vi "GeoData.vi"() -> ()   [LabVIEW 2017] (continued)
NJ\tBurlington County\tH1\n8022\t34005\tColumbus\tNJ\tBurlington County\tH1\n8060\t34005\tMount holly\tNJ\tBurlington County\tH1\n8640\t34005\tJoint base mdl\tNJ\tBurlington County\tH1\n8073\t34005\tRancocas\tNJ\tBurlington County\tH1\n8224\t34005\tNew gretna\tNJ\tBurlington County\tH1\n8043\t34005\tVoorhees\tNJ\tBurlington County\tH1\n8065\t34005\tPalmyra\tNJ\tBurlington County\tH1\n8052\t34005\tMaple shade\tNJ\tBurlington County\tH1\n8515\t34005\tChesterfield\tNJ\tBurlington County\tH1\n8046\t34005\tWillingboro\tNJ\tBurlington County\tH1\n8077\t34005\tRiverton\tNJ\tBurlington County\tH1\n8091\t34005\tWest berlin\tNJ\tBurlington County\tH1\n8641\t34005\tJoint base mdl\tNJ\tBurlington County\tH1\n8041\t34005\tJobstown\tNJ\tBurlington County\tH1\n8064\t34005\tNew lisbon\tNJ\tBurlington County\tH1\n8015\t34005\tBrowns mills\tNJ\tBurlington County\tH1\n8057\t34005\tMoorestown\tNJ\tBurlington County\tH1\n8087\t34005\tTuckerton\tNJ\tBurlington County\tH1\n8110\t34005\tPennsauken\tNJ\tBurlington County\tH1\n8215\t34005\tEgg harbor city\tNJ\tBurlington County\tH1\n8518\t34005\tFlorence\tNJ\tBurlington County\tH1\n8042\t34005\tJuliustown\tNJ\tBurlington County\tH1\n8053\t34005\tMarlton\tNJ\tBurlington County\tH1\n8054\t34005\tMount laurel\tNJ\tBurlington County\tH1\n8075\t34005\tRiverside\tNJ\tBurlington County\tH1\n8562\t34005\tWrightstown\tNJ\tBurlington County\tH1\n8620\t34005\tTrenton\tNJ\tBurlington County\tH1\n8011\t34005\tBirmingham\tNJ\tBurlington County\tH1\n8004\t34005\tAtco\tNJ\tBurlington County\tH1\n8010\t34005\tBeverly\tNJ\tBurlington County\tH1\n8048\t34005\tLumberton\tNJ\tBurlington County\tH1\n8088\t34005\tVincentown\tNJ\tBurlington County\tH1\n8068\t34005\tPemberton\tNJ\tBurlington County\tH1\n8016\t34005\tBurlington\tNJ\tBurlington County\tH1\n8055\t34005\tMedford\tNJ\tBurlington County\tH1\n8511\t34005\tCookstown\tNJ\tBurlington County\tH1\n8554\t34005\tRoebling\tNJ\tBurlington County\tH1\n8012\t34007\tBlackwood\tNJ\tCamden County\tH1\n8109\t34007\tMerchantville\tNJ\tCamden County\tH1\n8108\t34007\tCollingswood\tNJ\tCamden County\tH1\n8029\t34007\tGlendora\tNJ\tCamden County\tH1\n8002\t34007\tCherry hill\tNJ\tCamden County\tH1\n8037\t34007\tHammonton\tNJ\tCamden County\tH1\n8033\t34007\tHaddonfield\tNJ\tCamden County\tH1\n8049\t34007\tMagnolia\tNJ\tCamden County\tH1\n8081\t34007\tSicklerville\tNJ\tCamden County\tH1\n8035\t34007\tHaddon heights\tNJ\tCamden County\tH1\n8009\t34007\tBerlin\tNJ\tCamden County\tH1\n8043\t34007\tVoorhees\tNJ\tCamden County\tH1\n8065\t34007\tPalmyra\tNJ\tCamden County\tH1\n8052\t34007\tMaple shade\tNJ\tCamden County\tH1\n8080\t34007\tSewell\tNJ\tCamden County\tH1\n8084\t34007\tStratford\tNJ\tCamden County\tH1\n8106\t34007\tAudubon\tNJ\tCamden County\tH1\n8105\t34007\tCamden\tNJ\tCamden County\tH1\n8101\t34007\tCamden\tNJ\tCamden County\tH1\n8003\t34007\tCherry hill\tNJ\tCamden County\tH1\n8021\t34007\tClementon\tNJ\tCamden County\tH1\n8030\t34007\tGloucester city\tNJ\tCamden County\tH1\n8083\t34007\tSomerdale\tNJ\tCamden County\tH1\n8103\t34007\tCamden\tNJ\tCamden County\tH1\n8091\t34007\tWest berlin\tNJ\tCamden County\tH1\n8102\t34007\tCamden\tNJ\tCamden County\tH1\n8045\t34007\tLawnside\tNJ\tCamden County\tH1\n8110\t34007\tPennsauken\tNJ\tCamden County\tH1\n8099\t34007\tBellmawr\tNJ\tCamden County\tH1\n8095\t34007\tWinslow\tNJ\tCamden County\tH1\n8018\t34007\tCedar brook\tNJ\tCamden County\tH1\n8007\t34007\tBarrington\tNJ\tCamden County\tH1\n8026\t34007\tGibbsboro\tNJ\tCamden County\tH1\n8078\t34007\tRunnemede\tNJ\tCamden County\tH1\n8004\t34007\tAtco\tNJ\tCamden County\tH1\n8034\t34007\tCherry hill\tNJ\tCamden County\tH1\n8107\t34007\tOaklyn\tNJ\tCamden County\tH1\n8059\t34007\tMount ephraim\tNJ\tCamden County\tH1\n8104\t34007\tCamden\tNJ\tCamden County\tH1\n8089\t34007\tWaterford works\tNJ\tCamden County\tH1\n8031\t34007\tBellmawr\tNJ\tCamden County\tH1\n8223\t34009\tMarmora\tNJ\tCape May County\tH1\n8212\t34009\tCape may point\tNJ\tCape May County\tH1\n8248\t34009\tStrathmere\tNJ\tCape May County\tH1\n8260\t34009\tWildwood\tNJ\tCape May County\tH1\n8270\t34009\tWoodbine\tNJ\tCape May County\tH1\n8245\t34009\tSouth dennis\tNJ\tCape May County\tH1\n8204\t34009\tCape may\tNJ\tCape May County\tH1\n8202\t34009\tAvalon\tNJ\tCape May County\tH1\n8230\t34009\tOcean view\tNJ\tCape May County\tH1\n8214\t34009\tDennisville\tNJ\tCape May County\tH1\n8218\t34009\tGoshen\tNJ\tCape May County\tH1\n8210\t34009\tCape may court house\tNJ\tCape May County\tH1\n8246\t34009\tSouth seaville\tNJ\tCape May County\tH1\n8247\t34009\tStone harbor\tNJ\tCape May County\tH1\n8314\t34009\tDelmont\tNJ\tCape May County\tH1\n8226\t34009\tOcean city\tNJ\tCape May County\tH1\n8252\t34009\tWhitesboro\tNJ\tCape May County\tH1\n8251\t34009\tVillas\tNJ\tCape May County\tH1\n8242\t34009\tRio grande\tNJ\tCape May County\tH1\n8250\t34009\tTuckahoe\tNJ\tCape May County\tH1\n8243\t34009\tSea isle city\tNJ\tCape May County\tH1\n8219\t34009\tGreen creek\tNJ\tCape May County\tH1\n8353\t34011\tShiloh\tNJ\tCumberland County\tH1\n8340\t34011\tMilmay\tNJ\tCumberland County\tH1\n8324\t34011\tHeislerville\tNJ\tCumberland County\tH1\n8313\t34011\tDeerfield street\tNJ\tCumberland County\tH1\n8332\t34011\tMillville\tNJ\tCumberland County\tH1\n8302\t34011\tBridgeton\tNJ\tCumberland County\tH1\n8270\t34011\tWoodbine\tNJ\tCumberland County\tH1\n8361\t34011\tVineland\tNJ\tCumberland County\tH1\n8321\t34011\tFortescue\tNJ\tCumberland County\tH1\n8320\t34011\tFairton\tNJ\tCumberland County\tH1\n8345\t34011\tNewport\tNJ\tCumberland County\tH1\n8329\t34011\tMauricetown\tNJ\tCumberland County\tH1\n8311\t34011\tCedarville\tNJ\tCumberland County\tH1\n8349\t34011\tPort norris\tNJ\tCumberland County\tH1\n8348\t34011\tPort elizabeth\tNJ\tCumberland County\tH1\n8316\t34011\tDorchester\tNJ\tCumberland County\tH1\n8360\t34011\tVineland\tNJ\tCumberland County\tH1\n8314\t34011\tDelmont\tNJ\tCumberland County\tH1\n8327\t34011\tLeesburg\tNJ\tCumberland County\tH1\n8352\t34011\tRosenhayn\tNJ\tCumberland County\tH1\n8318\t34011\tElmer\tNJ\tCumberland County\tH1\n8310\t34011\tBuena\tNJ\tCumberland County\tH1\n8315\t34011\tDividing creek\tNJ\tCumberland County\tH1\n8323\t34011\tGreenwich\tNJ\tCumberland County\tH1\n8344\t34011\tNewfield\tNJ\tCumberland County\tH1\n8362\t34011\tVineland\tNJ\tCumberland County\tH1\n7040\t34013\tMaplewood\tNJ\tEssex County\tH1\n7052\t34013\tWest orange\tNJ\tEssex County\tH1\n7068\t34013\tRoseland\tNJ\tEssex County\tH1\n7102\t34013\tNewark\tNJ\tEssex County\tH1\n7114\t34013\tNewark\tNJ\tEssex County\tH1\n7108\t34013\tNewark\tNJ\tEssex County\tH1\n7109\t34013\tBelleville\tNJ\tEssex County\tH1\n7107\t34013\tNewark\tNJ\tEssex County\tH1\n7003\t34013\tBloomfield\tNJ\tEssex County\tH1\n7021\t34013\tEssex fells\tNJ\tEssex County\tH1\n7042\t34013\tMontclair\tNJ\tEssex County\tH1\n7106\t34013\tNewark\tNJ\tEssex County\tH1\n7044\t34013\tVerona\tNJ\tEssex County\tH1\n7050\t34013\tOrange\tNJ\tEssex County\tH1\n7104\t34013\tNewark\tNJ\tEssex County\tH1\n7101\t34013\tNewark\tNJ\tEssex County\tH1\n7088\t34013\tVauxhall\tNJ\tEssex County\tH1\n7009\t34013\tCedar grove\tNJ\tEssex County\tH1\n7039\t34013\tLivingston\tNJ\tEssex County\tH1\n7111\t34013\tIrvington\tNJ\tEssex County\tH1\n7201\t34013\tElizabeth\tNJ\tEssex County\tH1\n7017\t34013\tEast orange\tNJ\tEssex County\tH1\n7004\t34013\tFairfield\tNJ\tEssex County\tH1\n7041\t34013\tMillburn\tNJ\tEssex County\tH1\n7175\t34013\tNewark\tNJ\tEssex County\tH1\n7083\t34013\tUnion\tNJ\tEssex County\tH1\n7007\t34013\tCaldwell\tNJ\tEssex County\tH1\n7051\t34013\tOrange\tNJ\tEssex County\tH1\n7018\t34013\tEast orange\tNJ\tEssex County\tH1\n7043\t34013\tMontclair\tNJ\tEssex County\tH1\n7079\t34013\tSouth orange\tNJ\tEssex County\tH1\n7103\t34013\tNewark\tNJ\tEssex County\tH1\n7112\t34013\tNewark\tNJ\tEssex County\tH1\n7205\t34013\tHillside\tNJ\tEssex County\tH1\n7028\t34013\tGlen ridge\tNJ\tEssex County\tH1\n7006\t34013\tCaldwell\tNJ\tEssex County\tH1\n7019\t34013\tEast orange\tNJ\tEssex County\tH1\n7078\t34013\tShort hills\tNJ\tEssex County\tH1\n7110\t34013\tNutley\tNJ\tEssex County\tH1\n7105\t34013\tNewark\tNJ\tEssex County\tH1\n8012\t34015\tBlackwood\tNJ\tGloucester County\tH1\n8051\t34015\tMantua\tNJ\tGloucester County\tH1\n8098\t34015\tWoodstown\tNJ\tGloucester County\tH1\n8328\t34015\tMalaga\tNJ\tGloucester County\tH1\n8061\t34015\tMount royal\tNJ\tGloucester County\tH1\n8081\t34015\tSicklerville\tNJ\tGloucester County\tH1\n8085\t34015\tSwedesboro\tNJ\tGloucester County\tH1\n8096\t34015\tWoodbury\tNJ\tGloucester County\tH1\n8322\t34015\tFranklinville\tNJ\tGloucester County\tH1\n8312\t34015\tClayton\tNJ\tGloucester County\tH1\n8074\t34015\tRichwood\tNJ\tGloucester County\tH1\n8080\t34015\tSewell\tNJ\tGloucester County\tH1\n8071\t34015\tPitman\tNJ\tGloucester County\tH1\n8028\t34015\tGlassboro\tNJ\tGloucester County\tH1\n8063\t34015\tNational park\tNJ\tGloucester County\tH1\n8086\t34015\tThorofare\tNJ\tGloucester County\tH1\n8093\t34015\tWestville\tNJ\tGloucester County\tH1\n8097\t34015\tWoodbury heights\tNJ\tGloucester County\tH1\n8056\t34015\tMickleton\tNJ\tGloucester County\tH1\n8014\t34015\tBridgeport\tNJ\tGloucester County\tH1\n8094\t34015\tWilliamstown\tNJ\tGloucester County\tH1\n8360\t34015\tVineland\tNJ\tGloucester County\tH1\n8062\t34015\tMullica hill\tNJ\tGloucester County\tH1\n8343\t34015\tMonroeville\tNJ\tGloucester County\tH1\n8025\t34015\tEwan\tNJ\tGloucester County\tH1\n8020\t34015\tClarksboro\tNJ\tGloucester County\tH1\n8066\t34015\tPaulsboro\tNJ\tGloucester County\tH1\n8090\t34015\tWenonah\tNJ\tGloucester County\tH1\n8032\t34015\tGrenloch\tNJ\tGloucester County\tH1\n8027\t34015\tGibbstown\tNJ\tGloucester County\tH1\n8344\t34015\tNewfield\tNJ\tGloucester County\tH1\n8039\t34015\tHarrisonville\tNJ\tGloucester County\tH1\n7303\t34017\tJersey city\tNJ\tHudson County\tH1\n7087\t34017\tUnion city\tNJ\tHudson County\tH1\n7310\t34017\tJersey city\tNJ\tHudson County\tH1\n7002\t34017\tBayonne\tNJ\tHudson County\tH1\n7031\t34017\tNorth arlington\tNJ\tHudson County\tH1\n7047\t34017\tNorth bergen\tNJ\tHudson County\tH1\n7302\t34017\tJersey city\tNJ\tHudson County\tH1\n7311\t34017\tJersey city\tNJ\tHudson County\tH1\n7097\t34017\tJersey city\tNJ\tHudson County\tH1\n7093\t34017\tWest new york\tNJ\tHudson County\tH1\n7304\t34017\tJersey city\tNJ\tHudson County\tH1\n7030\t34017\tHoboken\tNJ\tHudson County\tH1\n7094\t34017\tSecaucus\tNJ\tHudson County\tH1\n7307\t34017\tJersey city\tNJ\tHudson County\tH1\n7096\t34017\tSecaucus\tNJ\tHudson County\tH1\n7099\t34017\tKearny\tNJ\tHudson County\tH1\n7032\t34017\tKearny\tNJ\tHudson County\tH1\n7029\t34017\tHarrison\tNJ\tHudson County\tH1\n7086\t34017\tWeehawken\tNJ\tHudson County\tH1\n7305\t34017\tJersey city\tNJ\tHudson County\tH1\n7306\t34017\tJersey city\tNJ\tHudson County\tH1\n7399\t34017\tJersey city\tNJ\tHudson County\tH1\n8833\t34019\tLebanon\tNJ\tHunterdon County\tH1\n7865\t34019\tPort murray\tNJ\tHunterdon County\tH1\n8801\t34019\tAnnandale\tNJ\tHunterdon County\tH1\n8559\t34019\tStockton\tNJ\tHunterdon County\tH1\n8551\t34019\tRingoes\tNJ\tHunterdon County\tH1\n7831\t34019\tChangewater\tNJ\tHunterdon County\tH1\n8803\t34019\tBaptistown\tNJ\tHunterdon County\tH1\n7830\t34019\tCalifon\tNJ\tHunterdon County\tH1\n8802\t34019\tAsbury\tNJ\tHunterdon County\tH1\n8558\t34019\tSkillman\tNJ\tHunterdon County\tH1\n8825\t34019\tFrenchtown\tNJ\tHunterdon County\tH1\n8848\t34019\tMilford\tNJ\tHunterdon County\tH1\n8804\t34019\tBloomsbury\tNJ\tHunterdon County\tH1\n8887\t34019\tThree bridges\tNJ\tHunterdon County\tH1\n8885\t34019\tStanton\tNJ\tHunterdon County\tH1\n8876\t34019\tSomerville\tNJ\tHunterdon County\tH1\n8530\t34019\tLambertville\tNJ\tHunterdon County\tH1\n8809\t34019\tClinton\tNJ\tHunterdon County\tH1\n8525\t34019\tHopewell\tNJ\tHunterdon County\tH1\n8867\t34019\tPittstown\tNJ\tHunterdon County\tH1\n8560\t34019\tTitusville\tNJ\tHunterdon County\tH1\n8868\t34019\tQuakertown\tNJ\tHunterdon County\tH1\n8888\t34019\tWhitehouse\tNJ\tHunterdon County\tH1\n7882\t34019\tWashington\tNJ\tHunterdon County\tH1\n8822\t34019\tFlemington\tNJ\tHunterdon County\tH1\n8889\t34019\tWhitehouse station\tNJ\tHunterdon County\tH1\n8827\t34019\tHampton\tNJ\tHunterdon County\tH1\n8556\t34019\tRosemont\tNJ\tHunterdon County\tH1\n8870\t34019\tReadington\tNJ\tHunterdon County\tH1\n8557\t34019\tSergeantsville\tNJ\tHunterdon County\tH1\n8829\t34019\tHigh bridge\tNJ\tHunterdon County\tH1\n8826\t34019\tGlen gardner\tNJ\tHunterdon County\tH1\n8858\t34019\tOldwick\tNJ\tHunterdon County\tH1\n8853\t34019\tNeshanic station\tNJ\tHunterdon County\tH1\n7979\t34019\tPottersville\tNJ\tHunterdon County\tH1\n8512\t34021\tCranbury\tNJ\tMercer County\tH1\n8501\t34021\tAllentown\tNJ\tMercer County\tH1\n8610\t34021\tTrenton\tNJ\tMercer County\tH1\n8542\t34021\tPrinceton\tNJ\tMercer County\tH1\n8628\t34021\tTrenton\tNJ\tMercer County\tH1\n8604\t34021\tTrenton\tNJ\tMercer County\tH1\n8601\t34021\tTrenton\tNJ\tMercer County\tH1\n8534\t34021\tPennington\tNJ\tMercer County\tH1\n8607\t34021\tTrenton\tNJ\tMercer County\tH1\n8540\t34021\tPrinceton\tNJ\tMercer County\tH1\n8558\t34021\tSkillman\tNJ\tMercer County\tH1\n8638\t34021\tTrenton\tNJ\tMercer County\tH1\n8648\t34021\tLawrence township\tNJ\tMercer County\tH1\n8515\t34021\tChesterfield\tNJ\tMercer County\tH1\n8543\t34021\tPrinceton\tNJ\tMercer County\tH1\n8602\t34021\tTrenton\tNJ\tMercer County\tH1\n8550\t34021\tPrinceton junction\tNJ\tMercer County\tH1\n8629\t34021\tTrenton\tNJ\tMercer County\tH1\n8544\t34021\tPrinceton\tNJ\tMercer County\tH1\n8530\t34021\tLambertville\tNJ\tMercer County\tH1\n8561\t34021\tWindsor\tNJ\tMercer County\tH1\n8520\t34021\tHightstown\tNJ\tMercer County\tH1\n8691\t34021\tTrenton\tNJ\tMercer County\tH1\n8618\t34021\tTrenton\tNJ\tMercer County\tH1\n8650\t34021\tTrenton\tNJ\tMercer County\tH1\n8606\t34021\tTrenton\tNJ\tMercer County\tH1\n8603\t34021\tTrenton\tNJ\tMercer County\tH1\n8608\t34021\tTrenton\tNJ\tMercer County\tH1\n8525\t34021\tHopewell\tNJ\tMercer County\tH1\n8619\t34021\tTrenton\tNJ\tMercer County\tH1\n8690\t34021\tTrenton\tNJ\tMercer County\tH1\n8620\t34021\tTrenton\tNJ\tMercer County\tH1\n8560\t34021\tTitusville\tNJ\tMercer County\tH1\n8605\t34021\tTrenton\tNJ\tMercer County\tH1\n8609\t34021\tTrenton\tNJ\tMercer County\tH1\n8611\t34021\tTrenton\tNJ\tMercer County\tH1\n8902\t34023\tNorth brunswick\tNJ\tMiddlesex County\tH1\n8882\t34023\tSouth river\tNJ\tMiddlesex County\tH1\n8512\t34023\tCranbury\tNJ\tMiddlesex County\tH1\n7067\t34023\tColonia\tNJ\tMiddlesex County\tH1\n7064\t34023\tPort reading\tNJ\tMiddlesex County\tH1\n8812\t34023\tDunellen\tNJ\tMiddlesex County\tH1\n7735\t34023\tKeyport\tNJ\tMiddlesex County\tH1\n8536\t34023\tPlainsboro\tNJ\tMiddlesex County\tH1\n8828\t34023\tHelmetta\tNJ\tMiddlesex County\tH1\n8903\t34023\tNew brunswick\tNJ\tMiddlesex County\tH1\n7008\t34023\tCarteret\tNJ\tMiddlesex County\tH1\n8816\t34023\tEast brunswick\tNJ\tMiddlesex County\tH1\n8830\t34023\tIselin\tNJ\tMiddlesex County\tH1\n8832\t34023\tKeasbey\tNJ\tMiddlesex County\tH1\n8857\t34023\tOld bridge\tNJ\tMiddlesex County\tH1\n7747\t34023\tMatawan\tNJ\tMiddlesex County\tH1\n8540\t34023\tPrinceton\tNJ\tMiddlesex County\tH1\n8863\t34023\tFords\tNJ\tMiddlesex County\tH1\n8855\t34023\tPiscataway\tNJ\tMiddlesex County\tH1\n8933\t34023\tNew brunswick\tNJ\tMiddlesex County\tH1\n7001\t34023\tAvenel\tNJ\tMiddlesex County\tH1\n8817\t34023\tEdison\tNJ\tMiddlesex County\tH1\n8820\t34023\tEdison\tNJ\tMiddlesex County\tH1\n8862\t34023\tPerth amboy\tNJ\tMiddlesex County\tH1\n8884\t34023\tSpotswood\tNJ\tMiddlesex County\tH1\n7095\t34023\tWoodbridge\tNJ\tMiddlesex County\tH1\n8810\t34023\tDayton\tNJ\tMiddlesex County\tH1\n8818\t34023\tEdison\tNJ\tMiddlesex County\tH1\n8852\t34023\tMonmouth junction\tNJ\tMiddlesex County\tH1\n8859\t34023\tParlin\tNJ\tMiddlesex County\tH1\n8904\t34023\tHighland park\tNJ\tMiddlesex County\tH1\n8520\t34023\tHightstown\tNJ\tMiddlesex County\tH1\n8805\t34023\tBound brook\tNJ\tMiddlesex County\tH1\n8854\t34023\tPiscataway\tNJ\tMiddlesex County\tH1\n8879\t34023\tSouth amboy\tNJ\tMiddlesex County\tH1\n7065\t34023\tRahway\tNJ\tMiddlesex County\tH1\n7080\t34023\tSouth plainfield\tNJ\tMiddlesex County\tH1\n8823\t34023\tFranklin park\tNJ\tMiddlesex County\tH1\n8824\t34023\tKendall park\tNJ\tMiddlesex County\tH1\n8850\t34023\tMilltown\tNJ\tMiddlesex County\tH1\n8861\t34023\tPerth amboy\tNJ\tMiddlesex County\tH1\n8872\t34023\tSayreville\tNJ\tMiddlesex County\tH1\n8901\t34023\tNew brunswick\tNJ\tMiddlesex County\tH1\n7721\t34023\tCliffwood\tNJ\tMiddlesex County\tH1\n7751\t34023\tMorganville\tNJ\tMiddlesex County\tH1\n7077\t34023\tSewaren\tNJ\tMiddlesex County\tH1\n8831\t34023\tMonroe township\tNJ\tMiddlesex County\tH1\n8840\t34023\tMetuchen\tNJ\tMiddlesex County\tH1\n8846\t34023\tMiddlesex\tNJ\tMiddlesex County\tH1\n8837\t34023\tEdison\tNJ\tMiddlesex County\tH1\n7726\t34023\tEnglishtown\tNJ\tMiddlesex County\tH1\n8528\t34023\tKingston\tNJ\tMiddlesex County\tH1\n8906\t34023\tNew brunswick\tNJ\tMiddlesex County\tH1\n8899\t34023\tEdison\tNJ\tMiddlesex County\tH1\n7727\t34025\tFarmingdale\tNJ\tMonmouth County\tH1\n7723\t34025\tDeal\tNJ\tMonmouth County\tH1\n7738\t34025\tLincroft\tNJ\tMonmouth County\tH1\n7754\t34025\tNeptune\tNJ\tMonmouth County\tH1\n7739\t34025\tLittle silver\tNJ\tMonmouth County\tH1\n8501\t34025\tAllentown\tNJ\tMonmouth County\tH1\n8736\t34025\tManasquan\tNJ\tMonmouth County\tH1\n7718\t34025\tBelford\tNJ\tMonmouth County\tH1\n7701\t34025\tRed bank\tNJ\tMonmouth County\tH1\n7712\t34025\tAsbury park\tNJ\tMonmouth County\tH1\n7732\t34025\tHighlands\tNJ\tMonmouth County\tH1\n7760\t34025\tRumson\tNJ\tMonmouth County\tH1\n7735\t34025\tKeyport\tNJ\tMonmouth County\tH1\n7764\t34025\tWest long branch\tNJ\tMonmouth County\tH1\n8514\t34025\tCream ridge\tNJ\tMonmouth County\tH1\n8527\t34025\tJackson\tNJ\tMonmouth County\tH1\n8750\t34025\tSea girt\tNJ\tMonmouth County\tH1\n7752\t34025\tNavesink\tNJ\tMonmouth County\tH1\n8555\t34025\tRoosevelt\tNJ\tMonmouth County\tH1\n7704\t34025\tFair haven\tNJ\tMonmouth County\tH1\n7728\t34025\tFreehold\tNJ\tMonmouth County\tH1\n7747\t34025\tMatawan\tNJ\tMonmouth County\tH1\n7746\t34025\tMarlboro\tNJ\tMonmouth County\tH1\n7762\t34025\tSpring lake\tNJ\tMonmouth County\tH1\n8730\t34025\tBrielle\tNJ\tMonmouth County\tH1\n7711\t34025\tAllenhurst\tNJ\tMonmouth County\tH1\n7710\t34025\tAdelphia\tNJ\tMonmouth County\tH1\n7731\t34025\tHowell\tNJ\tMonmouth County\tH1\n7740\t34025\tLong branch\tNJ\tMonmouth County\tH1\n7748\t34025\tMiddletown\tNJ\tMonmouth County\tH1\n8720\t34025\tAllenwood\tNJ\tMonmouth County\tH1\n7703\t34025\tFort monmouth\tNJ\tMonmouth County\tH1\n7733\t34025\tHolmdel\tNJ\tMonmouth County\tH1\n7719\t34025\tBelmar\tNJ\tMonmouth County\tH1\n7750\t34025\tMonmouth beach\tNJ\tMonmouth County\tH1\n8520\t34025\tHightstown\tNJ\tMonmouth County\tH1\n8535\t34025\tMillstone township\tNJ\tMonmouth County\tH1\n8691\t34025\tTrenton\tNJ\tMonmouth County\tH1\n7763\t34025\tTennent\tNJ\tMonmouth County\tH1\n7799\t34025\tEatontown\tNJ\tMonmouth County\tH1\n7724\t34025\tEatontown\tNJ\tMonmouth County\tH1\n7730\t34025\tHazlet\tNJ\tMonmouth County\tH1\n7737\t34025\tLeonardo\tNJ\tMonmouth County\tH1\n7757\t34025\tOceanport\tNJ\tMonmouth County\tH1\n7758\t34025\tPort monmouth\tNJ\tMonmouth County\tH1\n8562\t34025\tWrightstown\tNJ\tMonmouth County\tH1\n8620\t34025\tTrenton\tNJ\tMonmouth County\tH1\n7720\t34025\tBradley beach\tNJ\tMonmouth County\tH1\n7765\t34025\tWickatunk\tNJ\tMonmouth County\tH1\n7716\t34025\tAtlantic highlands\tNJ\tMonmouth County\tH1\n7721\t34025\tCliffwood\tNJ\tMonmouth County\tH1\n7751\t34025\tMorganville\tNJ\tMonmouth County\tH1\n7753\t34025\tNeptune\tNJ\tMonmouth County\tH1\n8510\t34025\tMillstone township\tNJ\tMonmouth County\tH1\n7755\t34025\tOakhurst\tNJ\tMonmouth County\tH1\n7702\t34025\tShrewsbury\tNJ\tMonmouth County\tH1\n7717\t34025\tAvon by the sea\tNJ\tMonmouth County\tH1\n7726\t34025\tEnglishtown\tNJ\tMonmouth County\tH1\n7734\t34025\tKeansburg\tNJ\tMonmouth County\tH1\n7722\t34025\tColts neck\tNJ\tMonmouth County\tH1\n7756\t34025\tOcean grove\tNJ\tMonmouth County\tH1\n8724\t34025\tBrick\tNJ\tMonmouth County\tH1\n7927\t34027\tCedar knolls\tNJ\tMorris County\tH1\n7457\t34027\tRiverdale\tNJ\tMorris County\tH1\n7935\t34027\tGreen village\tNJ\tMorris County\tH1\n7082\t34027\tTowaco\tNJ\tMorris County\tH1\n7405\t34027\tButler\tNJ\tMorris County\tH1\n7852\t34027\tLedgewood\tNJ\tMorris County\tH1\n7849\t34027\tLake hopatcong\tNJ\tMorris County\tH1\n7865\t34027\tPort murray\tNJ\tMorris County\tH1\n7936\t34027\tEast hanover\tNJ\tMorris County\tH1\n7933\t34027\tGillette\tNJ\tMorris County\tH1\n7932\t34027\tFlorham park\tNJ\tMorris County\tH1\n7930\t34027\tChester\tNJ\tMorris County\tH1\n7970\t34027\tMount freedom\tNJ\tMorris County\tH1\n7054\t34027\tParsippany\tNJ\tMorris County\tH1\n7403\t34027\tBloomingdale\tNJ\tMorris County\tH1\n7828\t34027\tBudd lake\tNJ\tMorris County\tH1\n7836\t34027\tFlanders\tNJ\tMorris County\tH1\n7830\t34027\tCalifon\tNJ\tMorris County\tH1\n7976\t34027\tNew vernon\tNJ\tMorris County\tH1\n7962\t34027\tMorristown\tNJ\tMorris County\tH1\n7058\t34027\tPine brook\tNJ\tMorris County\tH1\n7801\t34027\tDover\tNJ\tMorris County\tH1\n7850\t34027\tLanding\tNJ\tMorris County\tH1\n7866\t34027\tRockaway\tNJ\tMorris County\tH1\n7945\t34027\tMendham\tNJ\tMorris County\tH1\n7878\t34027\tMount tabor\tNJ\tMorris County\tH1\n7870\t34027\tSchooleys mountain\tNJ\tMorris County\tH1\n7034\t34027\tLake hiawatha\tNJ\tMorris County\tH1\n7940\t34027\tMadison\tNJ\tMorris County\tH1\n7926\t34027\tBrookside\tNJ\tMorris County\tH1\n7961\t34027\tConvent station\tNJ\tMorris County\tH1\n7845\t34027\tIronia\tNJ\tMorris County\tH1\n7005\t34027\tBoonton\tNJ\tMorris County\tH1\n7460\t34027\tStockholm\tNJ\tMorris County\tH1\n7834\t34027\tDenville\tNJ\tMorris County\tH1\n7856\t34027\tMount arlington\tNJ\tMorris County\tH1\n7847\t34027\tKenvil\tNJ\tMorris County\tH1\n7928\t34027\tChatham\tNJ\tMorris County\tH1\n7885\t34027\tWharton\tNJ\tMorris County\tH1\n7980\t34027\tStirling\tNJ\tMorris County\tH1\n7802\t34027\tDover\tNJ\tMorris County\tH1\n7857\t34027\tNetcong\tNJ\tMorris County\tH1\n7035\t34027\tLincoln park\tNJ\tMorris County\tH1\n7045\t34027\tMontville\tNJ\tMorris County\tH1\n7444\t34027\tPompton plains\tNJ\tMorris County\tH1\n7438\t34027\tOak ridge\tNJ\tMorris County\tH1\n7803\t34027\tMine hill\tNJ\tMorris County\tH1\n7869\t34027\tRandolph\tNJ\tMorris County\tH1\n7920\t34027\tBasking ridge\tNJ\tMorris County\tH1\n7960\t34027\tMorristown\tNJ\tMorris County\tH1\n7950\t34027\tMorris plains\tNJ\tMorris County\tH1\n7931\t34027\tFar hills\tNJ\tMorris County\tH1\n7924\t34027\tBernardsville\tNJ\tMorris County\tH1\n7981\t34027\tWhippany\tNJ\tMorris County\tH1\n7046\t34027\tMountain lakes\tNJ\tMorris County\tH1\n7963\t34027\tMorristown\tNJ\tMorris County\tH1\n7435\t34027\tNewfoundland\tNJ\tMorris County\tH1\n7853\t34027\tLong valley\tNJ\tMorris County\tH1\n7840\t34027\tHackettstown\tNJ\tMorris County\tH1\n7876\t34027\tSuccasunna\tNJ\tMorris County\tH1\n7946\t34027\tMillington\tNJ\tMorris County\tH1\n7934\t34027\tGladstone\tNJ\tMorris County\tH1\n7440\t34027\tPequannock\tNJ\tMorris County\tH1\n7806\t34027\tPicatinny arsenal\tNJ\tMorris County\tH1\n7842\t34027\tHibernia\tNJ\tMorris County\tH1\n8734\t34029\tLanoka harbor\tNJ\tOcean County\tH1\n8757\t34029\tToms river\tNJ\tOcean County\tH1\n8759\t34029\tManchester township\tNJ\tOcean County\tH1\n8758\t34029\tWaretown\tNJ\tOcean County\tH1\n8754\t34029\tToms river\tNJ\tOcean County\tH1\n8514\t34029\tCream ridge\tNJ\tOcean County\tH1\n8527\t34029\tJackson\tNJ\tOcean County\tH1\n8753\t34029\tToms river\tNJ\tOcean County\tH1\n8741\t34029\tPine beach\tNJ\tOcean County\tH1\n8739\t34029\tNormandy beach\tNJ\tOcean County\tH1\n7728\t34029\tFreehold\tNJ\tOcean County\tH1\n8006\t34029\tBarnegat light\tNJ\tOcean County\tH1\n7731\t34029\tHowell\tNJ\tOcean County\tH1\n8721\t34029\tBayville\tNJ\tOcean County\tH1\n8723\t34029\tBrick\tNJ\tOcean County\tH1\n8733\t34029\tLakehurst\tNJ\tOcean County\tH1\n8087\t34029\tTuckerton\tNJ\tOcean County\tH1\n8722\t34029\tBeachwood\tNJ\tOcean County\tH1\n8742\t34029\tPoint pleasant beach\tNJ\tOcean County\tH1\n8751\t34029\tSeaside heights\tNJ\tOcean County\tH1\n8731\t34029\tForked river\tNJ\tOcean County\tH1\n8752\t34029\tSeaside park\tNJ\tOcean County\tH1\n8732\t34029\tIsland heights\tNJ\tOcean County\tH1\n8701\t34029\tLakewood\tNJ\tOcean County\tH1\n8533\t34029\tNew egypt\tNJ\tOcean County\tH1\n8008\t34029\tBeach haven\tNJ\tOcean County\tH1\n8050\t34029\tManahawkin\tNJ\tOcean County\tH1\n8735\t34029\tLavallette\tNJ\tOcean County\tH1\n8740\t34029\tOcean gate\tNJ\tOcean County\tH1\n8755\t34029\tToms river\tNJ\tOcean County\tH1\n8005\t34029\tBarnegat\tNJ\tOcean County\tH1\n8092\t34029\tWest creek\tNJ\tOcean County\tH1\n8724\t34029\tBrick\tNJ\tOcean County\tH1\n8738\t34029\tMantoloking\tNJ\tOcean County\tH1\n7013\t34031\tClifton\tNJ\tPassaic County\tH1\n7012\t34031\tClifton\tNJ\tPassaic County\tH1\n7424\t34031\tLittle falls\tNJ\tPassaic County\tH1\n7508\t34031\tHaledon\tNJ\tPassaic County\tH1\n7522\t34031\tPaterson\tNJ\tPassaic County\tH1\n7474\t34031\tWayne\tNJ\tPassaic County\tH1\n7503\t34031\tPaterson\tNJ\tPassaic County\tH1\n7015\t34031\tClifton\tNJ\tPassaic County\tH1\n7421\t34031\tHewitt\tNJ\tPassaic County\tH1\n7403\t34031\tBloomingdale\tNJ\tPassaic County\tH1\n7506\t34031\tHawthorne\tNJ\tPassaic County\tH1\n7481\t34031\tWyckoff\tNJ\tPassaic County\tH1\n7507\t34031\tHawthorne\tNJ\tPassaic County\tH1\n7055\t34031\tPassaic\tNJ\tPassaic County\tH1\n7501\t34031\tPaterson\tNJ\tPassaic County\tH1\n7512\t34031\tTotowa\tNJ\tPassaic County\tH1\n7480\t34031\tWest milford\tNJ\tPassaic County\tH1\n7505\t34031\tPaterson\tNJ\tPassaic County\tH1\n7511\t34031\tTotowa\tNJ\tPassaic County\tH1\n7538\t34031\tHaledon\tNJ\tPassaic County\tH1\n7543\t34031\tPaterson\tNJ\tPassaic County\tH1\n7504\t34031\tPaterson\tNJ\tPassaic County\tH1\n7514\t34031\tPaterson\tNJ\tPassaic County\tH1\n7465\t34031\tWanaque\tNJ\tPassaic County\tH1\n7070\t34031\tRutherford\tNJ\tPassaic County\tH1\n7420\t34031\tHaskell\tNJ\tPassaic County\tH1\n7470\t34031\tWayne\tNJ\tPassaic County\tH1\n7460\t34031\tStockholm\tNJ\tPassaic County\tH1\n7524\t34031\tPaterson\tNJ\tPassaic County\tH1\n7442\t34031\tPompton lakes\tNJ\tPassaic County\tH1\n7510\t34031\tPaterson\tNJ\tPassaic County\tH1\n7014\t34031\tClifton\tNJ\tPassaic County\tH1\n7043\t34031\tMontclair\tNJ\tPassaic County\tH1\n7438\t34031\tOak ridge\tNJ\tPassaic County\tH1\n7513\t34031\tPaterson\tNJ\tPassaic County\tH1\n7509\t34031\tPaterson\tNJ\tPassaic County\tH1\n7544\t34031\tPaterson\tNJ\tPassaic County\tH1\n7006\t34031\tCaldwell\tNJ\tPassaic County\tH1\n7011\t34031\tClifton\tNJ\tPassaic County\tH1\n7110\t34031\tNutley\tNJ\tPassaic County\tH1\n7410\t34031\tFair lawn\tNJ\tPassaic County\tH1\n7435\t34031\tNewfoundland\tNJ\tPassaic County\tH1\n7456\t34031\tRingwood\tNJ\tPassaic County\tH1\n7502\t34031\tPaterson\tNJ\tPassaic County\tH1\n8079\t34033\tSalem\tNJ\tSalem County\tH1\n8098\t34033\tWoodstown\tNJ\tSalem County\tH1\n8023\t34033\tDeepwater\tNJ\tSalem County\tH1\n8085\t34033\tSwedesboro\tNJ\tSalem County\tH1\n8302\t34033\tBridgeton\tNJ\tSalem County\tH1\n8069\t34033\tPenns grove\tNJ\tSalem County\tH1\n8067\t34033\tPedricktown\tNJ\tSalem County\tH1\n8347\t34033\tNorma\tNJ\tSalem County\tH1\n8001\t34033\tAlloway\tNJ\tSalem County\tH1\n8070\t34033\tPennsville\tNJ\tSalem County\tH1\n8318\t34033\tElmer\tNJ\tSalem County\tH1\n8343\t34033\tMonroeville\tNJ\tSalem County\tH1\n8344\t34033\tNewfield\tNJ\tSalem County\tH1\n8038\t34033\tHancocks bridge\tNJ\tSalem County\tH1\n8072\t34033\tQuinton\tNJ\tSalem County\tH1\n7060\t34035\tPlainfield\tNJ\tSomerset County\tH1\n7921\t34035\tBedminster\tNJ\tSomerset County\tH1\n7978\t34035\tPluckemin\tNJ\tSomerset County\tH1\n8807\t34035\tBridgewater\tNJ\tSomerset County\tH1\n8812\t34035\tDunellen\tNJ\tSomerset County\tH1\n7076\t34035\tScotch plains\tNJ\tSomerset County\tH1\n7922\t34035\tBerkeley heights\tNJ\tSomerset County\tH1\n8875\t34035\tSomerset\tNJ\tSomerset County\tH1\n8540\t34035\tPrinceton\tNJ\tSomerset County\tH1\n8558\t34035\tSkillman\tNJ\tSomerset County\tH1\n7059\t34035\tWarren\tNJ\tSomerset County\tH1\n7945\t34035\tMendham\tNJ\tSomerset County\tH1\n8876\t34035\tSomerville\tNJ\tSomerset County\tH1\n8553\t34035\tRocky hill\tNJ\tSomerset County\tH1\n8835\t34035\tManville\tNJ\tSomerset County\tH1\n8502\t34035\tBelle mead\tNJ\tSomerset County\tH1\n7063\t34035\tPlainfield\tNJ\tSomerset County\tH1\n8805\t34035\tBound brook\tNJ\tSomerset County\tH1\n8836\t34035\tMartinsville\tNJ\tSomerset County\tH1\n8873\t34035\tSomerset\tNJ\tSomerset County\tH1\n8869\t34035\tRaritan\tNJ\tSomerset County\tH1\n8525\t34035\tHopewell\tNJ\tSomerset County\tH1\n8504\t34035\tBlawenburg\tNJ\tSomerset County\tH1\n7920\t34035\tBasking ridge\tNJ\tSomerset County\tH1\n7931\t34035\tFar hills\tNJ\tSomerset County\tH1\n7924\t34035\tBernardsville\tNJ\tSomerset County\tH1\n8822\t34035\tFlemington\tNJ\tSomerset County\tH1\n8823\t34035\tFranklin park\tNJ\tSomerset County\tH1\n8901\t34035\tNew brunswick\tNJ\tSomerset County\tH1\n8889\t34035\tWhitehouse station\tNJ\tSomerset County\tH1\n7069\t34035\tWatchung\tNJ\tSomerset County\tH1\n7938\t34035\tLiberty corner\tNJ\tSomerset County\tH1\n7939\t34035\tLyons\tNJ\tSomerset County\tH1\n7062\t34035\tPlainfield\tNJ\tSomerset County\tH1\n8844\t34035\tHillsborough\tNJ\tSomerset County\tH1\n8880\t34035\tSouth bound brook\tNJ\tSomerset County\tH1\n8528\t34035\tKingston\tNJ\tSomerset County\tH1\n7934\t34035\tGladstone\tNJ\tSomerset County\tH1\n8853\t34035\tNeshanic station\tNJ\tSomerset County\tH1\n8821\t34035\tFlagtown\tNJ\tSomerset County\tH1\n7977\t34035\tPeapack\tNJ\tSomerset County\tH1\n7871\t34037\tSparta\tNJ\tSussex County\tH1\n7839\t34037\tGreendell\tNJ\tSussex County\tH1\n7419\t34037\tHamburg\tNJ\tSussex County\tH1\n7439\t34037\tOgdensburg\tNJ\tSussex County\tH1\n7822\t34037\tAugusta\tNJ\tSussex County\tH1\n7860\t34037\tNewton\tNJ\tSussex County\tH1\n7849\t34037\tLake hopatcong\tNJ\tSussex County\tH1\n7851\t34037\tLayton\tNJ\tSussex County\tH1\n7879\t34037\tTranquility\tNJ\tSussex County\tH1\n7421\t34037\tHewitt\tNJ\tSussex County\tH1\n7422\t34037\tHighland lakes\tNJ\tSussex County\tH1\n7874\t34037\tStanhope\tNJ\tSussex County\tH1\n7837\t34037\tGlasser\tNJ\tSussex County\tH1\n7890\t34037\tBranchville\tNJ\tSussex County\tH1\n7418\t34037\tGlenwood\tNJ\tSussex County\tH1\n7416\t34037\tFranklin\tNJ\tSussex County\tH1\n7462\t34037\tVernon\tNJ\tSussex County\tH1\n7827\t34037\tMontague\tNJ\tSussex County\tH1\n7855\t34037\tMiddleville\tNJ\tSussex County\tH1\n7428\t34037\tMc afee\tNJ\tSussex County\tH1\n7821\t34037\tAndover\tNJ\tSussex County\tH1\n7826\t34037\tBranchville\tNJ\tSussex County\tH1\n7848\t34037\tLafayette\tNJ\tSussex County\tH1\n7460\t34037\tStockholm\tNJ\tSussex County\tH1\n7843\t34037\tHopatcong\tNJ\tSussex County\tH1\n7857\t34037\tNetcong\tNJ\tSussex County\tH1\n7461\t34037\tSussex\tNJ\tSussex County\tH1\n7832\t34037\tColumbia\tNJ\tSussex County\tH1\n7875\t34037\tStillwater\tNJ\tSussex County\tH1\n7877\t34037\tSwartswood\tNJ\tSussex County\tH1\n7825\t34037\tBlairstown\tNJ\tSussex County\tH1\n7036\t34039\tLinden\tNJ\tUnion County\tH1\n7040\t34039\tMaplewood\tNJ\tUnion County\tH1\n7060\t34039\tPlainfield\tNJ\tUnion County\tH1\n7114\t34039\tNewark\tNJ\tUnion County\tH1\n7204\t34039\tRoselle park\tNJ\tUnion County\tH1\n7974\t34039\tNew providence\tNJ\tUnion County\tH1\n7067\t34039\tColonia\tNJ\tUnion County\tH1\n8812\t34039\tDunellen\tNJ\tUnion County\tH1\n7061\t34039\tPlainfield\tNJ\tUnion County\tH1\n7023\t34039\tFanwood\tNJ\tUnion County\tH1\n7076\t34039\tScotch plains\tNJ\tUnion County\tH1\n7088\t34039\tVauxhall\tNJ\tUnion County\tH1\n7202\t34039\tElizabeth\tNJ\tUnion County\tH1\n7922\t34039\tBerkeley heights\tNJ\tUnion County\tH1\n7016\t34039\tCranford\tNJ\tUnion County\tH1\n7033\t34039\tKenilworth\tNJ\tUnion County\tH1\n7092\t34039\tMountainside\tNJ\tUnion County\tH1\n7111\t34039\tIrvington\tNJ\tUnion County\tH1\n7206\t34039\tElizabethport\tNJ\tUnion County\tH1\n7201\t34039\tElizabeth\tNJ\tUnion County\tH1\n7902\t34039\tSummit\tNJ\tUnion County\tH1\n8820\t34039\tEdison\tNJ\tUnion County\tH1\n7203\t34039\tRoselle\tNJ\tUnion County\tH1\n7027\t34039\tGarwood\tNJ\tUnion County\tH1\n7063\t34039\tPlainfield\tNJ\tUnion County\tH1\n7066\t34039\tClark\tNJ\tUnion County\tH1\n7081\t34039\tSpringfield\tNJ\tUnion County\tH1\n7083\t34039\tUnion\tNJ\tUnion County\tH1\n7208\t34039\tElizabeth\tNJ\tUnion County\tH1\n8854\t34039\tPiscataway\tNJ\tUnion County\tH1\n7091\t34039\tWestfield\tNJ\tUnion County\tH1\n7065\t34039\tRahway\tNJ\tUnion County\tH1\n7080\t34039\tSouth plainfield\tNJ\tUnion County\tH1\n7090\t34039\tWestfield\tNJ\tUnion County\tH1\n7205\t34039\tHillside\tNJ\tUnion County\tH1\n7207\t34039\tElizabeth\tNJ\tUnion County\tH1\n7901\t34039\tSummit\tNJ\tUnion County\tH1\n7069\t34039\tWatchung\tNJ\tUnion County\tH1\n7062\t34039\tPlainfield\tNJ\tUnion County\tH1\n7078\t34039\tShort hills\tNJ\tUnion County\tH1\n7880\t34041\tVienna\tNJ\tWarren County\tH1\n7860\t34041\tNewton\tNJ\tWarren County\tH1\n7865\t34041\tPort murray\tNJ\tWarren County\tH1\n7846\t34041\tJohnsonburg\tNJ\tWarren County\tH1\n7874\t34041\tStanhope\tNJ\tWarren County\tH1\n8802\t34041\tAsbury\tNJ\tWarren County\tH1\n8865\t34041\tPhillipsburg\tNJ\tWarren County\tH1\n8886\t34041\tStewartsville\tNJ\tWarren County\tH1\n8848\t34041\tMilford\tNJ\tWarren County\tH1\n8804\t34041\tBloomsbury\tNJ\tWarren County\tH1\n7838\t34041\tGreat meadows\tNJ\tWarren County\tH1\n7821\t34041\tAndover\tNJ\tWarren County\tH1\n8808\t34041\tBroadway\tNJ\tWarren County\tH1\n7863\t34041\tOxford\tNJ\tWarren County\tH1\n7820\t34041\tAllamuchy\tNJ\tWarren County\tH1\n7823\t34041\tBelvidere\tNJ\tWarren County\tH1\n7882\t34041\tWashington\tNJ\tWarren County\tH1\n7832\t34041\tColumbia\tNJ\tWarren County\tH1\n8827\t34041\tHampton\tNJ\tWarren County\tH1\n7844\t34041\tHope\tNJ\tWarren County\tH1\n7825\t34041\tBlairstown\tNJ\tWarren County\tH1\n7840\t34041\tHackettstown\tNJ\tWarren County\tH1\n7833\t34041\tDelaware\tNJ\tWarren County\tH1\n87110\t35001\tAlbuquerque\tNM\tBernalillo County\tH1\n87068\t35001\tBosque farms\tNM\tBernalillo County\tH1\n87035\t35001\tMoriarty\tNM\tBernalillo County\tH1\n87015\t35001\tEdgewood\tNM\tBernalillo County\tH1\n87103\t35001\tAlbuquerque\tNM\tBernalillo County\tH1\n87105\t35001\tAlbuquerque\tNM\tBernalillo County\tH1\n87047\t35001\tSandia park\tNM\tBernalillo County\tH1\n87048\t35001\tCorrales\tNM\tBernalillo County\tH1\n87176\t35001\tAlbuquerque\tNM\tBernalillo County\tH1\n87197\t35001\tAlbuquerque\tNM\tBernalillo County\tH1\n87190\t35001\tAlbuquerque\tNM\tBernalillo County\tH1\n87131\t35001\tAlbuquerque\tNM\tBernalillo County\tH1\n87108\t35001\tAlbuquerque\tNM\tBernalillo County\tH1\n87111\t35001\tAlbuquerque\tNM\tBernalillo County\tH1\n87122\t35001\tAlbuquerque\tNM\tBernalillo County\tH1\n87154\t35001\tAlbuquerque\tNM\tBernalillo County\tH1\n87008\t35001\tCedar crest\tNM\tBernalillo County\tH1\n87116\t35001\tAlbuquerque\tNM\tBernalillo County\tH1\n87109\t35001\tAlbuquerque\tNM\tBernalillo County\tH1\n87112\t35001\tAlbuquerque\tNM\tBernalillo County\tH1\n87113\t35001\tAlbuquerque\tNM\tBernalillo County\tH1\n87124\t35001\tRio rancho\tNM\tBernalillo County\tH1\n87121\t35001\tAlbuquerque\tNM\tBernalillo County\tH1\n87181\t35001\tAlbuquerque\tNM\tBernalillo County\tH1\n87199\t35001\tAlbuquerque\tNM\tBernalillo County\tH1\n87195\t35001\tAlbuquerque\tNM\tBernalillo County\tH1\n87187\t35001\tAlbuquerque\tNM\tBernalillo County\tH1\n87106\t35001\tAlbuquerque\tNM\tBernalillo County\tH1\n87120\t35001\tAlbuquerque\tNM\tBernalillo County\tH1\n87102\t35001\tAlbuquerque\tNM\tBernalillo County\tH1\n87101\t35001\tAlbuquerque\tNM\tBernalillo County\tH1\n87193\t35001\tAlbuquerque\tNM\tBernalillo County\tH1\n87119\t35001\tAlbuquerque\tNM\tBernalillo County\tH1\n87196\t35001\tAlbuquerque\tNM\tBernalillo County\tH1\n87153\t35001\tAlbuquerque\tNM\tBernalillo County\tH1\n87115\t35001\tAlbuquerque\tNM\tBernalillo County\tH1\n87104\t35001\tAlbuquerque\tNM\tBernalillo County\tH1\n87016\t35001\tEstancia\tNM\tBernalillo County\tH1\n87117\t35001\tKirtland afb\tNM\tBernalillo County\tH1\n87192\t35001\tAlbuquerque\tNM\tBernalillo County\tH1\n87022\t35001\tIsleta\tNM\tBernalillo County\tH1\n87059\t35001\tTijeras\tNM\tBernalillo County\tH1\n87144\t35001\tRio rancho\tNM\tBernalillo County\tH1\n87125\t35001\tAlbuquerque\tNM\tBernalillo County\tH1\n87184\t35001\tAlbuquerque\tNM\tBernalillo County\tH1\n87194\t35001\tAlbuquerque\tNM\tBernalillo County\tH1\n87185\t35001\tAlbuquerque\tNM\tBernalillo County\tH1\n87151\t35001\tAlbuquerque\tNM\tBernalillo County\tH1\n87114\t35001\tAlbuquerque\tNM\tBernalillo County\tH1\n87107\t35001\tAlbuquerque\tNM\tBernalillo County\tH1\n87123\t35001\tAlbuquerque\tNM\tBernalillo County\tH1\n87198\t35001\tAlbuquerque\tNM\tBernalillo County\tH1\n87191\t35001\tAlbuquerque\tNM\tBernalillo County\tH1\n87026\t35001\tLaguna\tNM\tBernalillo County\tH1\n87827\t35003\tPie town\tNM\tCatron County\tH1\n87829\t35003\tQuemado\tNM\tCatron County\tH1\n87820\t35003\tAragon\tNM\tCatron County\tH1\n87824\t35003\tLuna\tNM\tCatron County\tH1\n87830\t35003\tReserve\tNM\tCatron County\tH1\n87821\t35003\tDatil\tNM\tCatron County\tH1\n88039\t35003\tGlenwood\tNM\tCatron County\tH1\n88253\t35005\tLake arthur\tNM\tChaves County\tH1\n88232\t35005\tHagerman\tNM\tChaves County\tH1\n88201\t35005\tRoswell\tNM\tChaves County\tH1\n88250\t35005\tHope\tNM\tChaves County\tH1\n88344\t35005\tPinon\tNM\tChaves County\tH1\n88203\t35005\tRoswell\tNM\tChaves County\tH1\n88202\t35005\tRoswell\tNM\tChaves County\tH1\n88116\t35005\tElida\tNM\tChaves County\tH1\n88339\t35005\tMayhill\tNM\tChaves County\tH1\n88230\t35005\tDexter\tNM\tChaves County\tH1\n87020\t35006\tGrants\tNM\tCibola County\tH1\n87038\t35006\tNew laguna\tNM\tCibola County\tH1\n87323\t35006\tThoreau\tNM\tCibola County\tH1\n87040\t35006\tPaguate\tNM\tCibola County\tH1\n87357\t35006\tPinehill\tNM\tCibola County\tH1\n87049\t35006\tSan fidel\tNM\tCibola County\tH1\n87315\t35006\tFence lake\tNM\tCibola County\tH1\n87051\t35006\tSan rafael\tNM\tCibola County\tH1\n87007\t35006\tCasa blanca\tNM\tCibola County\tH1\n87005\t35006\tBluewater\tNM\tCibola County\tH1\n87034\t35006\tPueblo of acoma\tNM\tCibola County\tH1\n87045\t35006\tPrewitt\tNM\tCibola County\tH1\n87014\t35006\tCubero\tNM\tCibola County\tH1\n87021\t35006\tMilan\tNM\tCibola County\tH1\n87747\t35007\tSpringer\tNM\tColfax County\tH1\n87728\t35007\tMaxwell\tNM\tColfax County\tH1\n87718\t35007\tEagle nest\tNM\tColfax County\tH1\n87729\t35007\tMiami\tNM\tColfax County\tH1\n87752\t35007\tWagon mound\tNM\tColfax County\tH1\n88422\t35007\tGladstone\tNM\tColfax County\tH1\n88419\t35007\tFolsom\tNM\tColfax County\tH1\n87714\t35007\tCimarron\tNM\tColfax County\tH1\n87710\t35007\tAngel fire\tNM\tColfax County\tH1\n87740\t35007\tRaton\tNM\tColfax County\tH1\n87749\t35007\tUte park\tNM\tColfax County\tH1\n88124\t35009\tMelrose\tNM\tCurry County\tH1\n88102\t35009\tClovis\tNM\tCurry County\tH1\n88103\t35009\tCannon afb\tNM\tCurry County\tH1\n88120\t35009\tGrady\tNM\tCurry County\tH1\n88101\t35009\tClovis\tNM\tCurry County\tH1\n88130\t35009\tPortales\tNM\tCurry County\tH1\n88427\t35009\tMcalister\tNM\tCurry County\tH1\n88133\t35009\tSaint vrain\tNM\tCurry County\tH1\n88135\t35009\tTexico\tNM\tCurry County\tH1\n88118\t35009\tFloyd\tNM\tCurry County\tH1\n88112\t35009\tBroadview\tNM\tCurry County\tH1\n88119\t35011\tFort sumner\tNM\tDe Baca County\tH1\n88136\t35011\tYeso\tNM\tDe Baca County\tH1\n88081\t35013\tChaparral\tNM\tDona Ana County\tH1\n88005\t35013\tLas cruces\tNM\tDona Ana County\tH1\n88004\t35013\tLas cruces\tNM\tDona Ana County\tH1\n88027\t35013\tChamberino\tNM\tDona Ana County\tH1\n88007\t35013\tLas cruces\tNM\tDona Ana County\tH1\n88044\t35013\tLa mesa\tNM\tDona Ana County\tH1\n88063\t35013\tSunland park\tNM\tDona Ana County\tH1\n87940\t35013\tRincon\tNM\tDona Ana County\tH1\n88054\t35013\tRadium springs\tNM\tDona Ana County\tH1\n88021\t35013\tAnthony\tNM\tDona Ana County\tH1\n88047\t35013\tMesilla park\tNM\tDona Ana County\tH1\n87937\t35013\tHatch\tNM\tDona Ana County\t
